vi "Configure Module.vi"(8 "error in (no error)":errorcluster, 10 "IOV ref in":variant, 11 "Module Template in":refnum<class "Module Template.lvclass">) -> (0 "error out":errorcluster, 2 "IOV ref out":variant, 3 "Module Template out":refnum<class "Module Template.lvclass">)   [LabVIEW 2019, in "Modules.lvlib" / "Module Template.lvclass"]
uses:
  Module Template.lvclass
  <resource>/objmgr/cRIO.rc
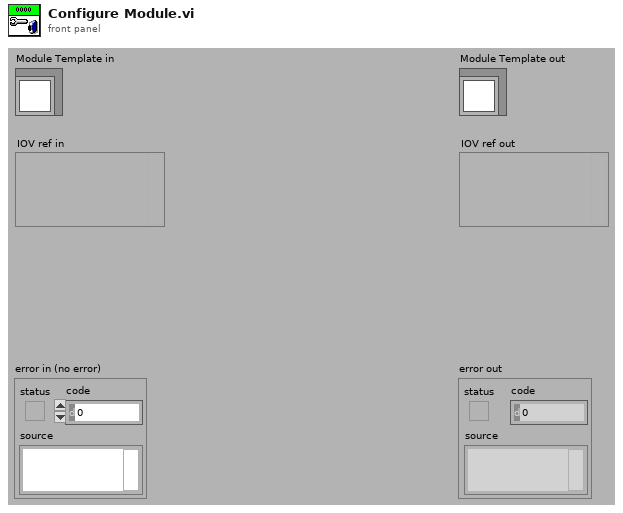
[diagram p1: front panel]
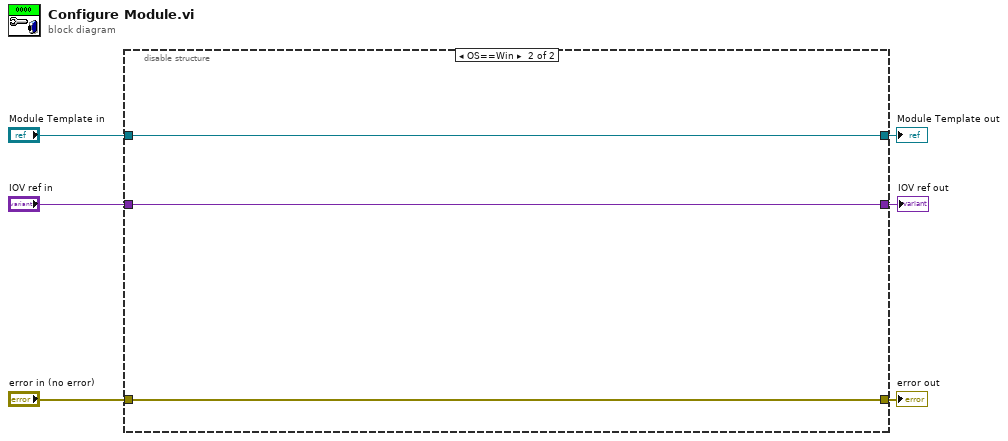
[diagram p0: block diagram]
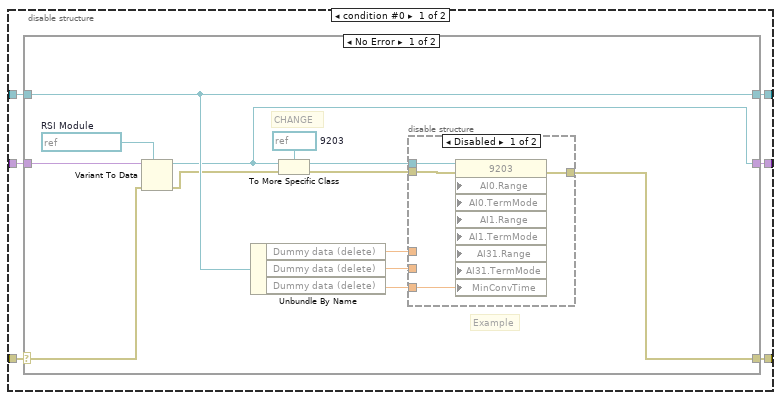
[diagram p2: hidden frame]
diagram:
  n1 = disable-structure shown="OS==Win" {
    disable-tunnel: "error in (no error)" -> [w12 w34]
    disable-tunnel: [w11 w34] -> w5
    disable-tunnel: "Module Template in" -> [w10 w36]
    disable-tunnel: [w9 w36] -> w3
    disable-tunnel: "IOV ref in" -> [w8 w35]
    disable-tunnel: [w7 w35] -> w1
    frame condition #0 {
      n2 = case shown="No Error" w12 {
        selector: w12 -> [w15 w33]
        tunnel: [w20 w33] -> w11
        tunnel: [w24 w32] -> w9
        tunnel: w10 -> [w24 w32]
        tunnel: w8 -> [w17 w31]
        tunnel: [w16 w31] -> w7
        frame No Error {
          w13 = refnum<k21> refnum  # RSI Module
          w23 = refnum<k21> refnum  # 9203
          # "CHANGE"
          # "Example"
          n3 = Variant To Data(error in=w15, type=w13, Variant=w17) -> (data=w16:refnum<k21>, error out=w14:errorcluster)
          n4 = Unbundle By Name(w24) -> ("Dummy data (delete)"=w19:dbl, "Dummy data (delete)"=w18:dbl, "Dummy data (delete)"=w25:dbl)
          n5 = To More Specific Class(target class=w23, reference=w16, error in=w14) -> (specific class reference=w22:refnum<k21>, error out=w21:errorcluster)
          n6 = disable-structure shown="Disabled" {
            disable-tunnel: w25 -> [w29 _]
            disable-tunnel: w22 -> [w28 _]
            disable-tunnel: w21 -> [w27 w30]
            disable-tunnel: [w26 w30] -> w20
            disable-tunnel: w19 -> [_ _]
            disable-tunnel: w18 -> [_ _]
            frame Disabled {
              n7 = property class="9203" props=["AI0.Range", "AI0.TermMode", "AI1.Range", "AI1.TermMode", "AI31.Range", "AI31.TermMode", "MinConvTime"](reference=w28, error in=w27, "MinConvTime"=w29) -> (error out=w26:errorcluster)  [unwired: 6 in, 1 out]
            }
            frame Enabled {
            }
          }
        }
        frame Error {
        }
      }
    }
    frame condition #1 (active) {
    }
  }
  "error out" <- w5
  "Module Template out" <- w3
  "IOV ref out" <- w1
